vi "Loops and Memory.vi"() -> ()   [LabVIEW 2019]
panel:
  in  "Button":bool
  out "millisecond timer value":u32
  out "Shift Register Value":dbl
  out "Out of Loop Indicator":dbl
  out "In Loop Indicator":dbl
  out "Numeric":i32
  in  "stop":bool
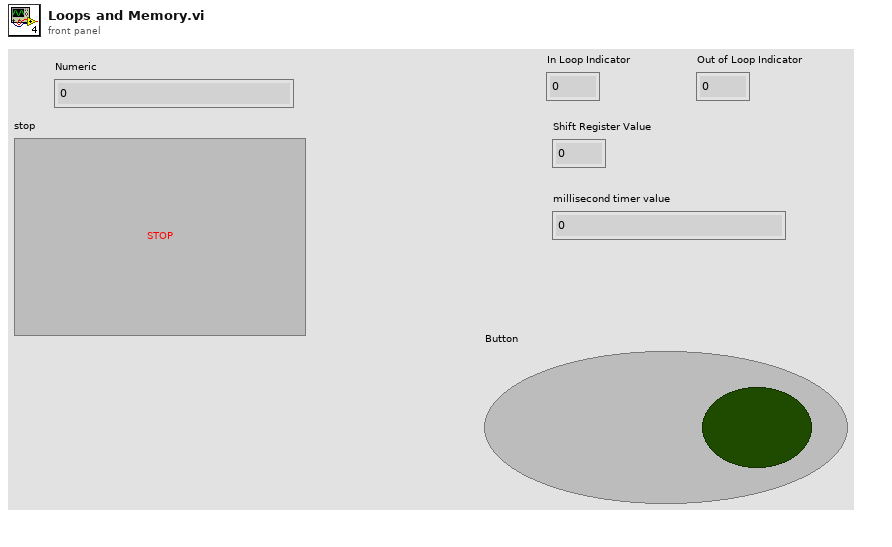
[diagram p1: front panel]
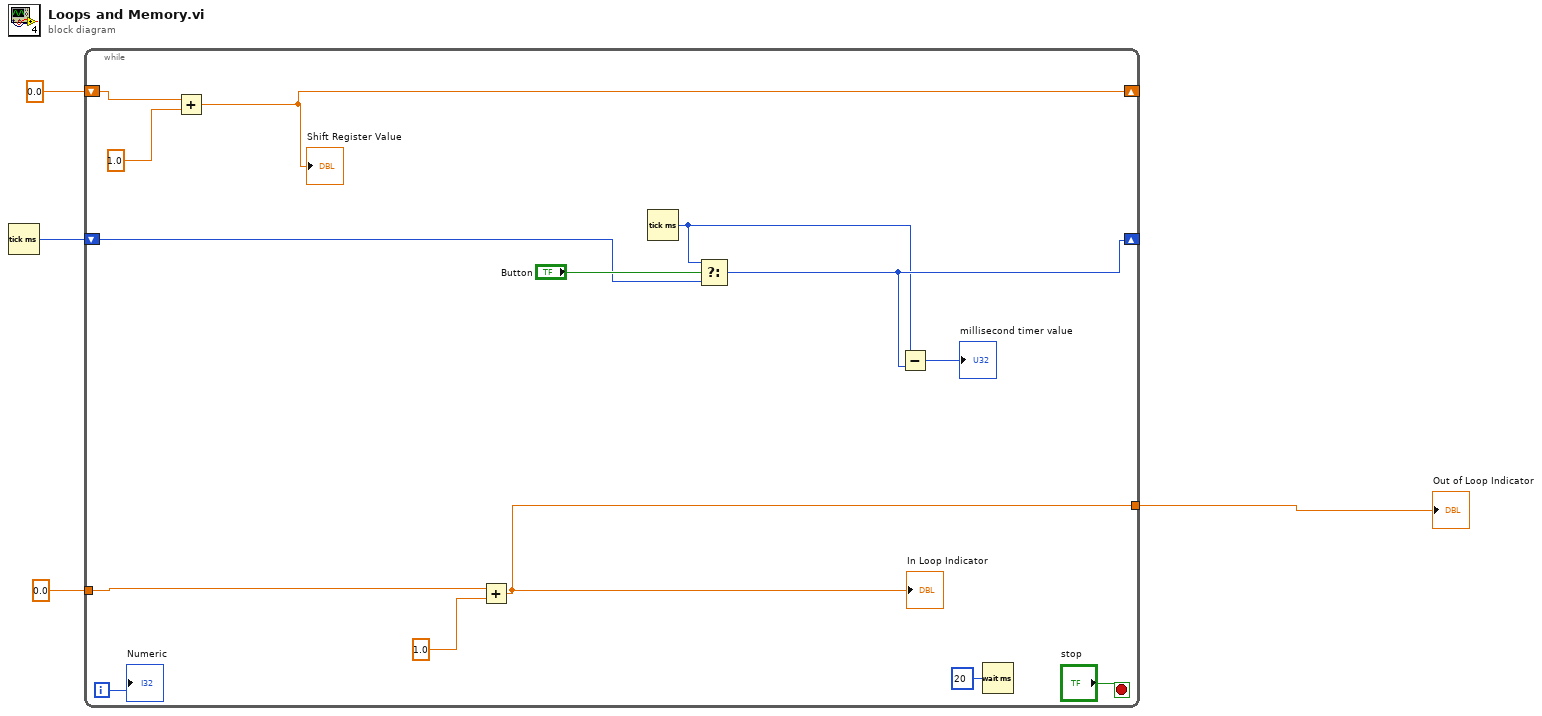
[diagram p0: block diagram]
diagram:
  n1 = Tick Count (ms)() -> (millisecond timer value=w1:u32)
  n2 = while {
    tunnel: [w14] -> w4
    tunnel: 0.0 -> [w13]
    shift-right: [w10] -> _
    shift-left: 0.0 -> [w11]
    shift-right: [w6] -> _
    shift-left: w1 -> [w7]
    i -> [w17]
    stop <- "stop" stop-if-true
    n3 = Add(x=w11, y=1.0) -> (x+y=w10:dbl)
    "Shift Register Value" <- w10
    n4 = Add(x=w13, y=1.0) -> (x+y=w14:dbl)
    "In Loop Indicator" <- w14
    n5 = Tick Count (ms)() -> (millisecond timer value=w5:u32)
    n6 = Select(t=w5, s="Button", f=w7) -> (s? t:f=w6:u32)
    n7 = Subtract(x=w5, y=w6) -> (x-y=→"millisecond timer value":u32)
    n8 = Wait (ms)(milliseconds to wait=u32 20) -> ()  [unwired: 1 out]
    "Numeric" <- w17
  }
  "Out of Loop Indicator" <- w4
